vi "Delete Sheet.vi"(8 "error in":errorcluster, 10 "Sheet Name":string, 11 "Worksheets 2":refnum<k7>) -> (0 "error out":errorcluster, 1 "Work Sheet":refnum<k7>, 2 "Worksheets":refnum<k7>)   [LabVIEW 2017]
panel:
  in  "Excel._Worksheet":refnum<k7>
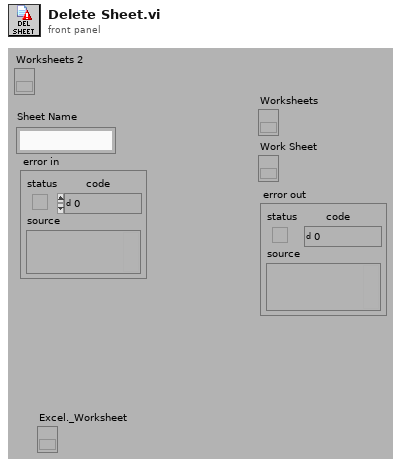
[diagram p1: front panel]
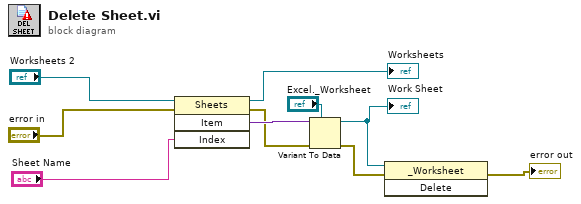
[diagram p0: block diagram]
diagram:
  n1 = invoke class="Sheets" method="Item"(reference="Worksheets 2", error in="error in", "Index"="Sheet Name") -> (reference out=→"Worksheets":refnum<k7>, error out=w9:errorcluster, "Item"=w10:variant)  [unwired: 1 in, 1 out]
  n2 = Variant To Data(error in=w9, type="Excel._Worksheet", Variant=w10) -> (data=w3:refnum<k7>, error out=w2:errorcluster)
  "Work Sheet" <- w3
  n3 = invoke class="_Worksheet" method="Delete"(reference=w3, error in=w2) -> (error out=→"error out":errorcluster)  [unwired: 1 in, 2 out]
